vi "NiSwitch CanConnect.vi"(6 "contextId":T1, 8 "error in":errorcluster, 9 "timeout (ms)":i32=-1, 10 "Request Data":T4, 11 "gRPC ID":T1) -> (0 "error out":errorcluster, 2 "Response Data":T2, 3 "gRPC ID out":T1)   [LabVIEW 2021, in "NI Switch_client.lvlib"]
uses:
  NI Switch_client.lvlib
  <vilib>/gRPC/LabVIEW gRPC Library/Shared/grpcId.ctl
  RPC Messages/niswitch_grpc_CanConnectRequest.ctl
  RPC Messages/nidevice_grpc_Session.ctl
  RPC Messages/niswitch_grpc_CanConnectResponse.ctl
  RPC Messages/niswitch_grpc_PathCapability.ctl
  RPC Messages/niswitch_grpc_CanConnectResponse_Flat.ctl
  14035477-4c25-4107-8ed5-d0c4ef420ce5.vi
  RPC Messages/RichToFlatnidevice_grpc_Session.vi
  <vilib>/gRPC/LabVIEW gRPC Library/Shared/TranslateGrpcError.vi
  <vilib>/gRPC/LabVIEW gRPC Library/Shared/Wait On Occurrence Wrapper.vi
  <vilib>/gRPC/LabVIEW gRPC Library/Shared/Wait On Occurence.vi
  <vilib>/gRPC/LabVIEW gRPC Library/Server API/Server/Get Server DLL Path.vi
  <vilib>/Utility/error.llb/Error Cluster From Error Code.vi
  <vilib>/Utility/config.llb/Open Config Data.vi
  <vilib>/Utility/config.llb/Write Key.vi
  <vilib>/Utility/config.llb/Write Key (Boolean).vi
  <vilib>/Utility/config.llb/Not A Config Data Refnum.vi
  <vilib>/Utility/config.llb/Read Key.vi
  <vilib>/Utility/config.llb/Read Key (Boolean).vi
  <vilib>/Utility/config.llb/Close Config Data.vi
  <vilib>/gRPC/LabVIEW gRPC Library/grpc-lvsupport-release.lvlib
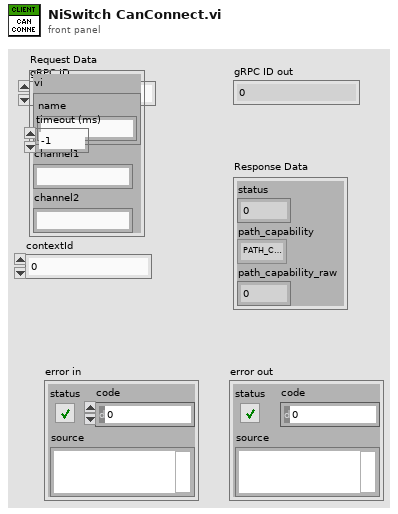
[diagram p1: front panel]
types:
  T1 = typedef "grpc-lvsupport-release.lvlib/grpcId.ctl" = u64
  T2 = typedef "NI Switch_client.lvlib/niswitch_grpc_CanConnectResponse.ctl" = cluster{"status":i32, "path_capability":T3, "path_capability_raw":i32}
  T3 = typedef "NI Switch_client.lvlib/niswitch_grpc_PathCapability.ctl" = enum32{"PATH_CAPABILITY_UNSPECIFIED", "PATH_CAPABILITY_NISWITCH_VAL_PATH_AVAILABLE", "PATH_CAPABILITY_NISWITCH_VAL_PATH_EXISTS", "PATH_CAPABILITY_NISWITCH_VAL_PATH_UNSUPPORTED", "PATH_CAPABILITY_NISWITCH_VAL_RESOURCE_IN_USE", "PATH_CAPABILITY_NISWITCH_VAL_SOURCE_CONFLICT", "PATH_CAPABILITY_NISWITCH_VAL_CHANNEL_NOT_AVAILABLE"}
  T4 = typedef "NI Switch_client.lvlib/niswitch_grpc_CanConnectRequest.ctl" = cluster{"vi":T5, "channel1":string, "channel2":string}
  T5 = typedef "NI Switch_client.lvlib/nidevice_grpc_Session.ctl" = cluster{"name":string}
  T6 = typedef "NI Switch_client.lvlib/niswitch_grpc_CanConnectResponse_Flat.ctl" = cluster{"status":i32, "path_capability":T3, "path_capability_raw":i32}
  T7 = typedef "NI Switch_client.lvlib/niswitch_grpc_CanConnectRequest_Flat.ctl" = cluster{"vi":T8, "channel1":string, "channel2":string}
  T8 = typedef "NI Switch_client.lvlib/nidevice_grpc_Session_Flat.ctl" = cluster{"name":string}
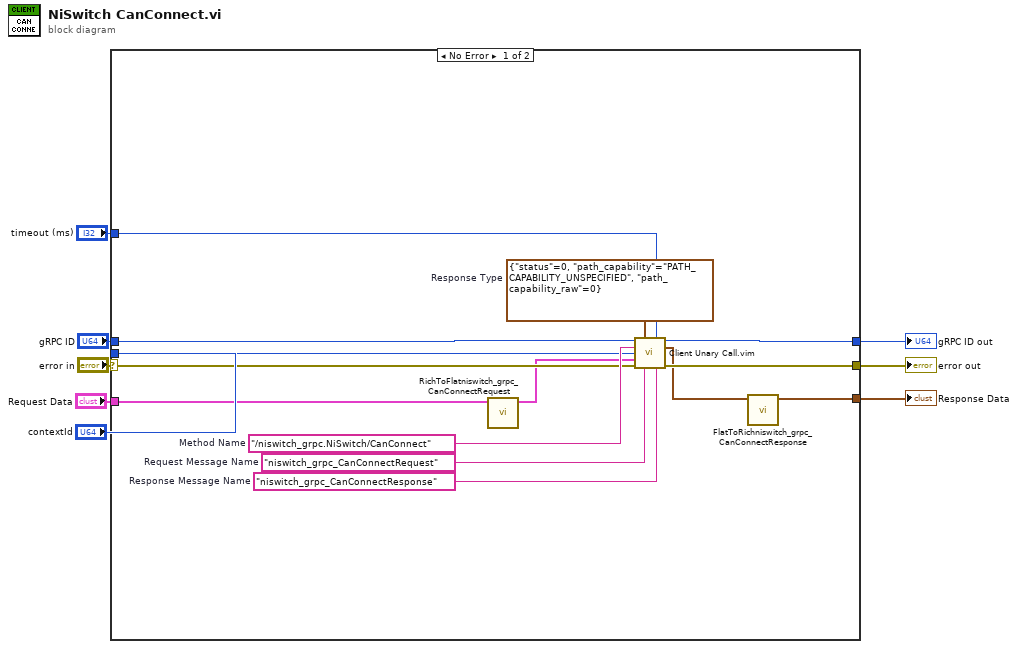
[diagram p0: block diagram]
diagram:
  n1 = case shown="No Error" "error in" {
    selector: "error in" -> [w18 w23]
    tunnel: [w17 w23] -> w7
    tunnel: "gRPC ID" -> [w16 w24]
    tunnel: [w15 w24] -> w5
    tunnel: "Request Data" -> [w12 _]
    tunnel: [w9 _] -> w3
    tunnel: "timeout (ms)" -> [w14 _]
    tunnel: "contextId" -> [w13 _]
    frame No Error {
      w19 = "niswitch_grpc_CanConnectResponse"  # Response Message Name
      w20 = "niswitch_grpc_CanConnectRequest"  # Request Message Name
      w21 = T6 {"status"=0, "path_capability"=enum."PATH_CAPABILITY_UNSPECIFIED", "path_capability_raw"=0}  # Response Type
      w22 = "/niswitch_grpc.NiSwitch/CanConnect"  # Method Name
      n2 = call "RichToFlatniswitch_grpc_CanConnectRequest.vi"("InputCluster"=w12) -> ("OutputCluster"=w11:T7)  [unwired: 10 in]
      n3 = call "Client Unary Call.vim"("ClientID in"=w16, "Response Type"=w21, "timeout (ms)"=w14, "Method Name"=w22, "contextId"=w13, "Request Data"=w11, "error in"=w18, "Request Message Name"=w20, "Response Message Name"=w19) -> ("ClientID out"=w15:u64, "Response Data"=w10:T6, "error out"=w17:errorcluster)  [unwired: 4 in]
      n4 = call "FlatToRichniswitch_grpc_CanConnectResponse.vi"("InputCluster"=w10) -> ("OutputCluster"=w9:T2)  [unwired: 10 in]
    }
    frame Error {
    }
  }
  "error out" <- w7
  "gRPC ID out" <- w5
  "Response Data" <- w3
